vi "Swerve Drive.vi"(0 "X":dbl(slide)=0.5 scale=-1.0..1.0, 3 "Y":dbl(slide) scale=1.0..-1.0, 6 "Z":dbl(knob) scale=1.0..-1.0, 10 "Rot. Point Y":dbl, 13 "Robot-Centric":bool, 16 "Rot. Point X":dbl) -> (20 "Back Left Spin Power":dbl=-0.0, 21 "Back Right Spin Power":dbl=-0.0, 22 "Front Left Spin Power":dbl=-0.0, 23 "Front Right Spin Power":dbl=-0.0, 24 "Back Left Motor Power":dbl=-0.59, 25 "Back Right Motor Power":dbl=0.5, 26 "Front Left Motor Power":dbl=0.59, 27 "Front Right Motor Power":dbl=-0.5)   [LabVIEW 2016]
doc: "Main block for a swerve drive. X, Y, and Z are the only inputs that must be wired.\nX and Y are the joystick axes for translational (strafing) movement. Z is the joystick axis for rotation. Rotation point is the point relative to the center of the robot (in inches), around which the robot rotates. This input is optional, leave it blank to always rotate around the center of the robot. If Auto Controls is true, then the inputs will not be squared, and there will be no deadband. If Robot-Centric is true, then the gyro will be ignored, and pushing forward on the joystick will result in a foward movement relative to the robot's direction."
uses:
  Drive Globals.vi
panel:
  in  "Robot Length":dbl=27.0
  in  "Robot Width":dbl=41.0
  # "SWERVE DRIVE\nVersion 3.1\n\nCory Lynch\nApple Pi Robotics\nTeam 2067"
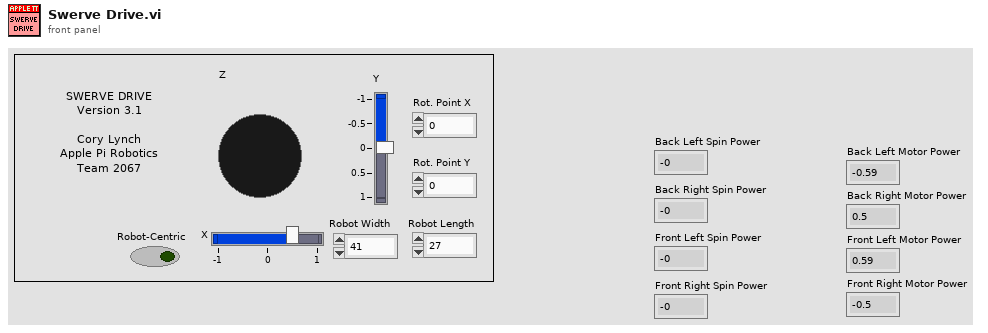
[diagram p1: front panel]
types:
  T1 = enum16{"Back Left", "Back Right", "Front Left", "Front Right"}
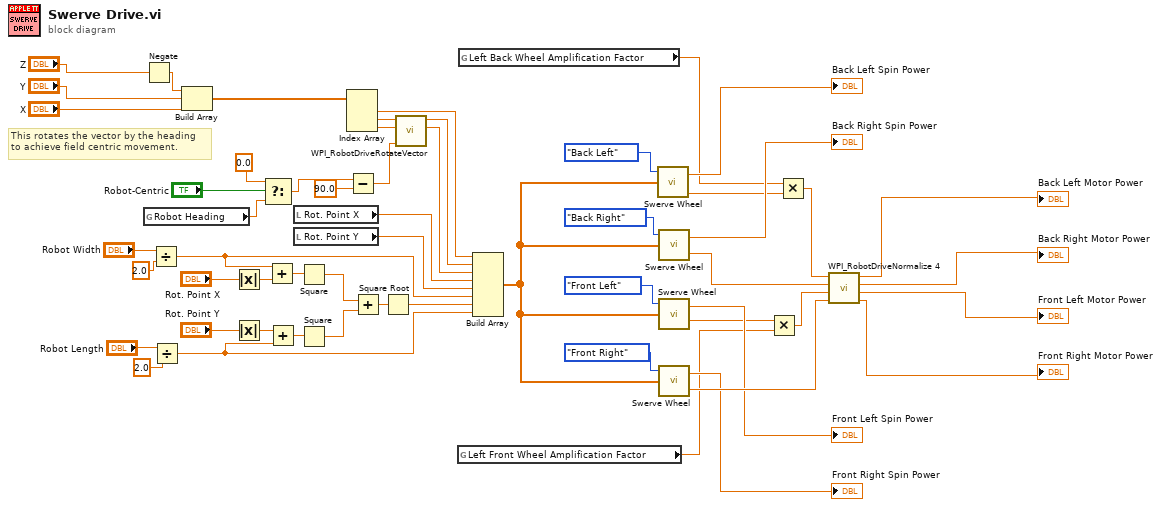
[diagram p0: block diagram]
diagram:
  # "This rotates the vector by the heading\nto achieve field centric movement."
  n1 = Negate(x="Z") -> (-x=w5:dbl)
  n2 = global read "Drive Globals.vi" "Robot Heading"() -> (w6:dbl)
  n3 = Divide(x="Robot Width", y=2.0) -> (x/y=w38:dbl)
  n4 = Divide(x="Robot Length", y=2.0) -> (x/y=w36:dbl)
  n5 = Build Array(w5, "Y", "X") -> (w1:dbl[])
  n6 = Absolute Value(x="Rot. Point X") -> (abs(x)=w54:dbl)
  n7 = Absolute Value(x="Rot. Point Y") -> (abs(x)=w52:dbl)
  n8 = Select(t=0.0, s="Robot-Centric", f=w6) -> (s? t:f=w17:dbl)
  n9 = Add(x=w38, y=w54) -> (x+y=w53:dbl)
  n10 = Add(x=w52, y=w36) -> (x+y=w51:dbl)
  n11 = local read "Rot. Point X"() -> (w40:dbl)
  n12 = local read "Rot. Point Y"() -> (w39:dbl)
  n13 = Square(x=w53) -> (x^2=w49:dbl)
  n14 = Square(x=w51) -> (x^2=w50:dbl)
  n15 = Index Array(array=w1) -> (element #1=w30:dbl, element #2=w35:dbl, element #3=w41:dbl)  [unwired: 3 in]
  n16 = Subtract(x=w17, y=90.0) -> (x-y=w16:dbl)
  n17 = Add(x=w49, y=w50) -> (x+y=w48:dbl)
  n18 = Square Root(x=w48) -> (sqrt(x)=w37:dbl)
  n19 = call <vilib>:"WPI_RobotDriveRotateVector.vi"("Angle"=w16, "X"=w41, "Y"=w35) -> ("X'"=w33:dbl, "Y'"=w29:dbl)  [unwired: 7 out]
  n20 = global read "Drive Globals.vi" "Left Front Wheel Amplification Factor"() -> (w8:dbl)
  n21 = global read "Drive Globals.vi" "Left Back Wheel Amplification Factor"() -> (w7:dbl)
  n22 = Build Array(w30, w29, w33, w40, w39, w38, w37, w36) -> (w34:dbl[])
  n23 = call "Swerve Wheel.vi"("Inputs"=w34, "Wheel"=T1."Back Left") -> ("Speed"=w9:dbl, "Spin Motor Power"=→"Back Left Spin Power":dbl)  [unwired: 2 in]
  n24 = call "Swerve Wheel.vi"("Inputs"=w34, "Wheel"=T1."Back Right") -> ("Speed"=w24:dbl, "Spin Motor Power"=→"Back Right Spin Power":dbl)  [unwired: 2 in]
  n25 = call "Swerve Wheel.vi"("Inputs"=w34, "Wheel"=T1."Front Left") -> ("Speed"=w10:dbl, "Spin Motor Power"=→"Front Left Spin Power":dbl)  [unwired: 2 in]
  n26 = call "Swerve Wheel.vi"("Inputs"=w34, "Wheel"=T1."Front Right") -> ("Speed"=w55:dbl, "Spin Motor Power"=→"Front Right Spin Power":dbl)  [unwired: 2 in]
  n27 = Multiply(x=w10, y=w8) -> (x*y=w11:dbl)
  n28 = Multiply(x=w7, y=w9) -> (x*y=w12:dbl)
  n29 = call <vilib>:"WPI_RobotDriveNormalize 4.vi"("D"=w55, "C"=w11, "B"=w24, "A"=w12) -> ("D'"=→"Front Right Motor Power":dbl, "C'"=→"Front Left Motor Power":dbl, "B'"=→"Back Right Motor Power":dbl, "A'"=→"Back Left Motor Power":dbl)
